vi "FileIntialize.vi"(8 "Error In":errorcluster, 9 "Delimeter":string, 10 "Labels":string[](array[string]), 11 "refnum in":refnum<file>) -> (0 "Error Out":errorcluster, 3 "File Refnum":refnum<file>)   [LabVIEW 2021]
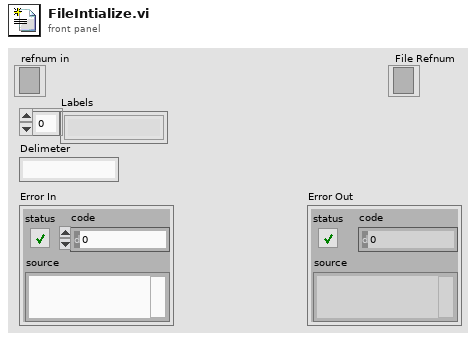
[diagram p1: front panel]
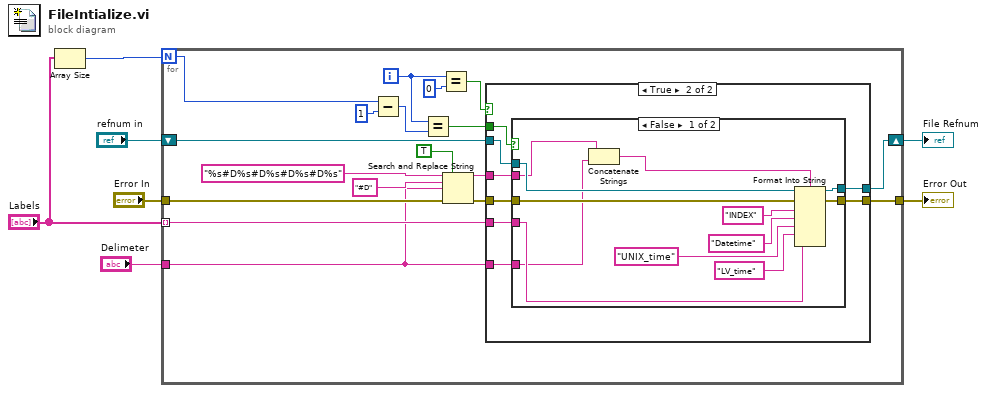
[diagram p0: block diagram]
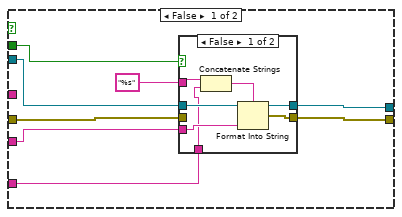
[diagram p2: hidden frame]
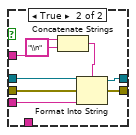
[diagram p3: hidden frame]
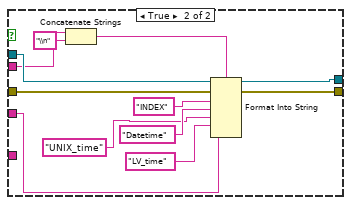
[diagram p4: hidden frame]
diagram:
  n1 = Array Size(array="Labels") -> (size(s)=w6:i32)
  n2 = for {
    N: w6 -> [w18]
    tunnel: [w20] -> w5
    tunnel: "Labels" -> [w19] mode=indexing
    tunnel: "Error In" -> [w11]
    shift-right: [w15] -> w4
    shift-left: "refnum in" -> [w25]
    tunnel: "Delimeter" -> [w8]
    i -> [w22]
    n3 = Subtract(x=w18, y=1 ("x")) -> (x-y=w17:i32)
    n4 = Equal?(x=w22, y=w17) -> (x = y?=w21:bool)
    n5 = Equal?(x=w22, y=0) -> (x = y?=w23:bool)
    n6 = Search and Replace String(replace all?=TRUE ("replace all? (F)"), input string="%s#D%s#D%s#D%s#D%s" ("format string"), search string="#D" ("format string"), replace string=w8, error in=w11) -> (result string=w9:string, error out=w10:errorcluster)  [unwired: 3 in, 2 out]
    n7 = case shown="True" w23 {
      tunnel: w25 -> [w33 w56]
      tunnel: w21 -> [w32 w55]
      tunnel: [w31 w53] -> w20
      tunnel: [w30 w54] -> w15
      tunnel: w19 -> [w29 w52]
      tunnel: w10 -> [w28 w51]
      tunnel: w9 -> [_ w50]
      tunnel: w8 -> [w26 w49]
      frame False {
        n8 = case shown="False" w32 {
          tunnel: w33 -> [w40 w48]
          tunnel: [w39 w47] -> w31
          tunnel: [w38 w46] -> w30
          tunnel: w29 -> [w37 w45]
          tunnel: w28 -> [_ w44]
          tunnel: "%s" ("format string") -> [w36 w43]
          tunnel: w26 -> [w35 _]
          frame False {
            n9 = Concatenate Strings(w36, w35) -> (w34:string)
            n10 = Format Into String(format string=w34, initial string=w40, w37) -> (resulting string=w38:refnum<file>, error out=w39:errorcluster)  [unwired: 1 in]
          }
          frame True {
            n11 = Concatenate Strings(w43, "\\n" ("string")) -> (w41:string)
            n12 = Format Into String(format string=w41, initial string=w48, error in=w44, w45) -> (resulting string=w46:refnum<file>, error out=w47:errorcluster)
          }
        }
      }
      frame True {
        n13 = case shown="False" w55 {
          tunnel: w56 -> [w64 w80]
          tunnel: [w62 w75] -> w54
          tunnel: [w63 w74] -> w53
          tunnel: w52 -> [w61 w73]
          tunnel: w51 -> [w60 w72]
          tunnel: w50 -> [w59 w71]
          tunnel: w49 -> [w58 _]
          frame False {
            n14 = Concatenate Strings(w59, w58) -> (w57:string)
            n15 = Format Into String(format string=w57, initial string=w64, error in=w60, "INDEX" ("input 1"), "Datetime" ("input 1"), "UNIX_time" ("input 1"), "LV_time" ("input 1"), w61) -> (resulting string=w62:refnum<file>, error out=w63:errorcluster)
          }
          frame True {
            n16 = Concatenate Strings(w71, "\\n" ("string")) -> (w69:string)
            n17 = Format Into String(format string=w69, initial string=w80, error in=w72, "INDEX" ("input 1"), "Datetime" ("input 1"), "UNIX_time" ("input 1"), "LV_time" ("input 1"), w73) -> (resulting string=w75:refnum<file>, error out=w74:errorcluster)
          }
        }
      }
    }
  }
  "File Refnum" <- w4
  "Error Out" <- w5
